vi "Read triangles from stl file (binary format).vi"(0 "STL file path":path=path "C:/EnFlo Software/Anemometry/Anemometry Sub Vis/Collision_Detection/Triangles/Example files/SR-71_Blackbird.STL") -> (1 "Triangles array":T1[](array[typedef]), 2 "N triangles":u32=3528, 3 "Error out":errorcluster)   [LabVIEW 2018]
doc: "Note: The STL file must be in binary format, not ASCII."
uses:
  Typedefs/Triangle.ctl
  Subroutines/Cross product 3D.vi
  Subroutines/Unit vector.vi
  Subroutines/Dot product.vi
panel:
  out "STL header":string
  # "PN 19/01/2015"
  # "Vertices"
  # "Edges"
  # "Unit normal"
  # "Edge unit normals"
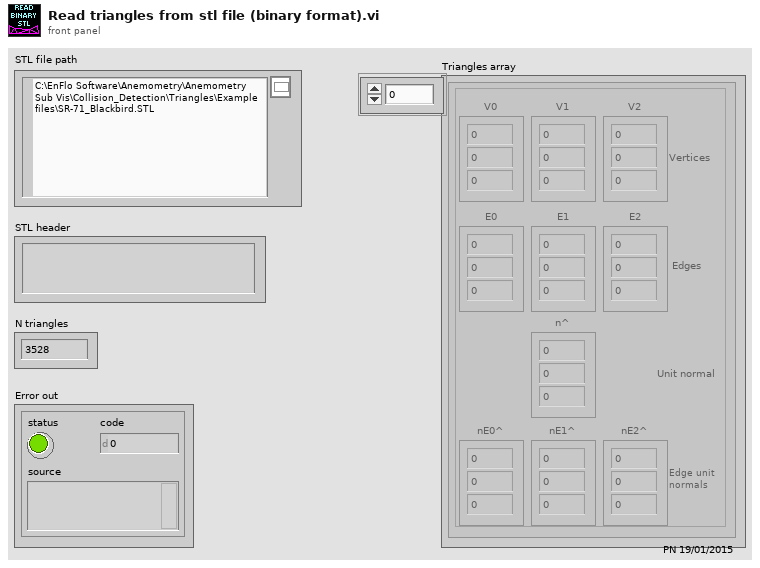
[diagram p1: front panel]
types:
  T1 = typedef "Triangle.ctl" = cluster{"V0":sgl[], "V1":sgl[], "V2":sgl[], "E0":sgl[], "E1":sgl[], "E2":sgl[], "n^":sgl[], "nE0^":sgl[], "nE1^":sgl[], "nE2^":sgl[]}
  T2 = enum16{"open", "replace", "create", "open or create", "replace or create", "replace or create with confirmation"}
  T3 = enum16{"big-endian, network order", "native, host order", "little-endian"}
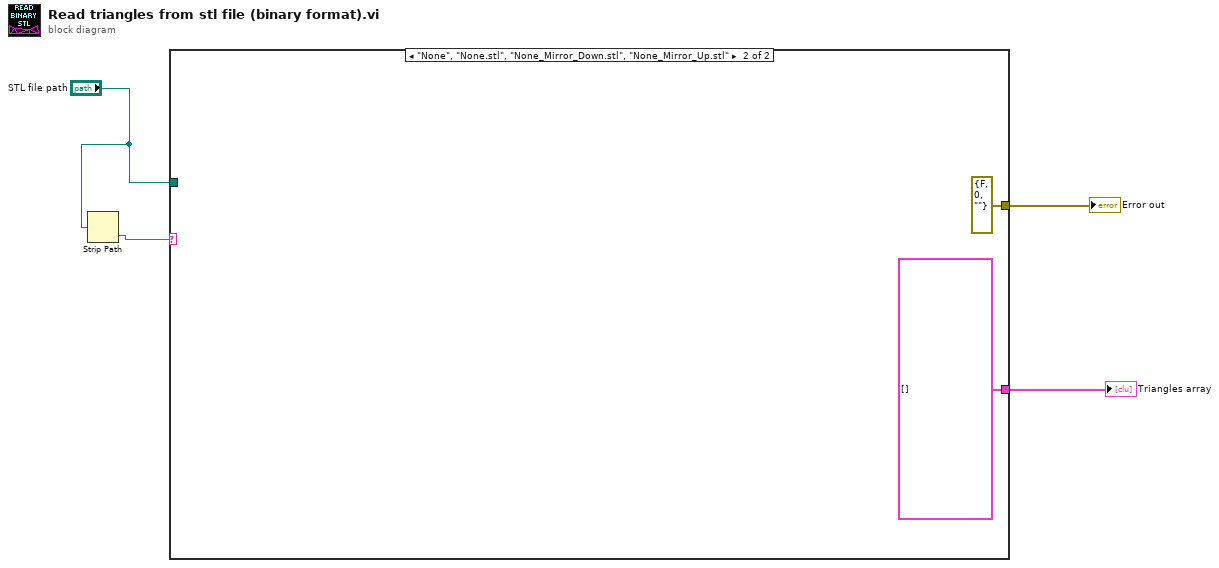
[diagram p0: block diagram]
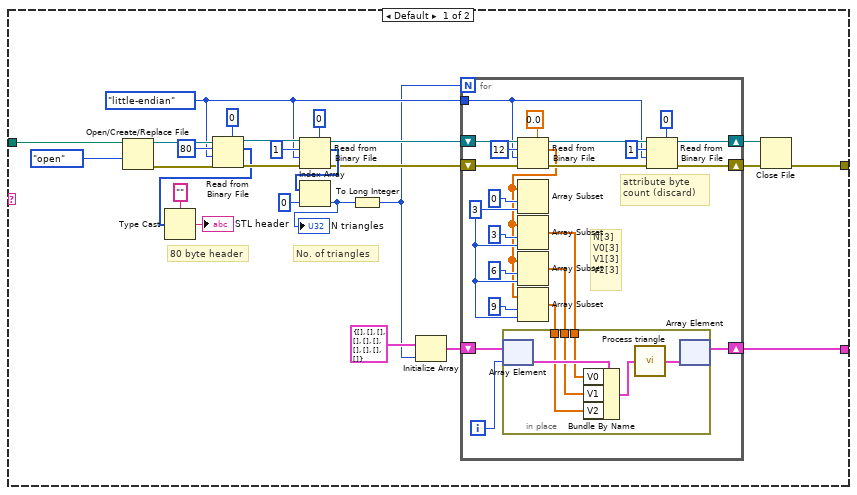
[diagram p2: hidden frame]
diagram:
  n1 = Strip Path(path="STL file path") -> (name=w1:string)  [unwired: 1 out]
  n2 = case shown="\"None\", \"None.stl\", \"None_Mirror_Down.stl\", \"None_Mirror_Up.stl\"" w1 {
    tunnel: [w12 errorcluster {"status"=FALSE, "code"=0, "source"=""} ("error out")] -> w4
    tunnel: [w6 T1[] []] -> w3
    tunnel: "STL file path" -> [w5 _]
    frame Default {
      w8 = T3."little-endian" ("byte order (0:big-endian, network order)")
      # "No. of triangles"
      # "80 byte header"
      n3 = Open/Create/Replace File(file path (use dialog)=w5, operation (0:open)=T2."open") -> (refnum out=w29:refnum<file>, error out=w28:errorcluster)  [unwired: 4 in, 1 out]
      n4 = Read from Binary File(5:u8 0, 8:w28, 9:w8, 10:80 ("count (1)"), 11:w29) -> (0:w21:errorcluster, 2:w19:u8[], 3:w23:refnum<file>)  [unwired: 1 in, 1 out]
      n5 = Type Cast(type="", x=w19) -> (*(type *) &x=→"STL header":string)
      n6 = Read from Binary File(5:u32 0, 8:w21, 9:w8, 10:1 ("count (1)"), 11:w23) -> (0:w16:errorcluster, 2:w18:u32[], 3:w15:refnum<file>)  [unwired: 1 in, 1 out]
      n7 = Index Array(array=w18, index=0) -> (element=w17:u32)
      "N triangles" <- w17
      n8 = To Long Integer(number=w17) -> (32bit integer=w7:i32)
      n9 = Initialize Array(T1 {"V0"=[], "V1"=[], "V2"=[], "E0"=[], "E1"=[], "E2"=[], "n^"=[], "nE0^"=[], "nE1^"=[], "nE2^"=[]} ("Cluster"), w7) -> (w10:T1[])
      n10 = for {
        N: w7 -> [_]
        shift-right: [w44] -> w13
        shift-left: w16 -> [w52]
        shift-right: [w45] -> w14
        shift-left: w15 -> [w53]
        shift-right: [w42] -> w6
        shift-left: w10 -> [w43]
        tunnel: w8 -> [w32]
        i -> [w31]
        w37 = 3 ("length")
        # "N[3]\nV0[3]\nV1[3]\nV2[3]"
        # "attribute byte count (discard)"
        n11 = Read from Binary File(5:sgl 0.0, 8:w52, 9:w32, 10:12 ("count (1)"), 11:w53) -> (0:w47:errorcluster, 2:w36:sgl[], 3:w46:refnum<file>)  [unwired: 1 in, 1 out]
        n12 = Array Subset(array=w36, index=0, length=w37) -> ()  [unwired: 1 out]
        n13 = Array Subset(array=w36, index=3, length=w37) -> (w35:sgl[])
        n14 = Array Subset(array=w36, index=6, length=w37) -> (w34:sgl[])
        n15 = Array Subset(array=w36, index=9, length=w37) -> (w33:sgl[])
        n16 = in-place {
          in-place-border: w35 -> [w56]
          in-place-border: w34 -> [w55]
          in-place-border: w33 -> [w54]
          n17 = in-place-array #1(w43, w31) -> (w58:T1)
          n18 = Bundle By Name(cluster=w58, "V0"=w56, "V1"=w55, "V2"=w54) -> (w57:T1)
          n19 = call "Process triangle.vi"("Triangle in"=w57) -> ("Triangle out"=w59:T1)
          n20 = in-place-array #1(w59) -> (w42:T1[])  [unwired: 1 out]
        }
        n21 = Read from Binary File(5:u16 0, 8:w47, 9:w32, 10:1 ("count (1)"), 11:w46) -> (0:w44:errorcluster, 3:w45:refnum<file>)  [unwired: 1 in, 2 out]
      }
      n22 = Close File(refnum=w14, error in=w13) -> (error out=w12:errorcluster)  [unwired: 1 out]
    }
    frame "None", "None.stl", "None_Mirror_Down.stl", "None_Mirror_Up.stl" {
    }
  }
  "Error out" <- w4
  "Triangles array" <- w3
